vi "FileSaveFile.vi"(0 "VISA IN":refnum<visa-resource-name>, 5 "error in":errorcluster) -> (14 "VISA Out":refnum<visa-resource-name>, 19 "error out":errorcluster)   [LabVIEW 2018, in "PNA-X.lvlib"]
uses:
  PNA-X.lvlib
panel:
  in  "Type":string(combo)
  in  "Port numbers":string
  in  "File":string
  in  "Combo Box":string(combo)="CSA"
  in  "Channel":i32=1
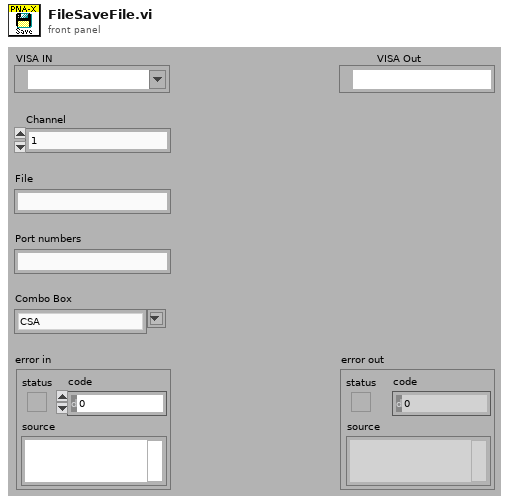
[diagram p1: front panel]
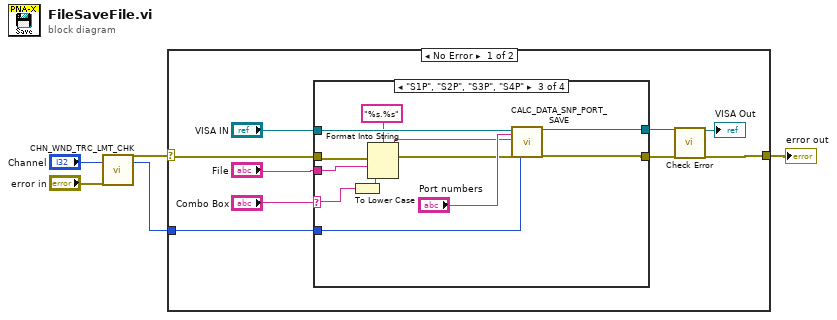
[diagram p0: block diagram]
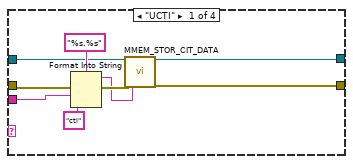
[diagram p2: hidden frame]
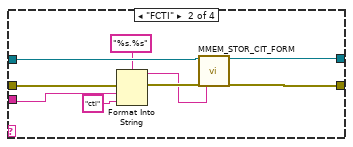
[diagram p3: hidden frame]
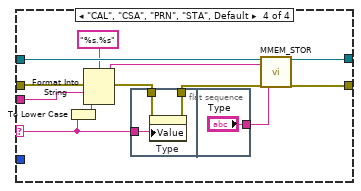
[diagram p4: hidden frame]
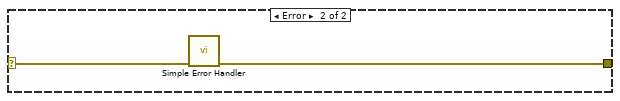
[diagram p5: hidden frame]
diagram:
  n1 = call "CHN_WND_TRC_LMT_CHK.vi"("Channel"="Channel", "error in"="error in") -> ("error out"=w2:errorcluster, "Channel"=w1:i32)  [unwired: 13 in, 3 out]
  n2 = case shown="No Error" w2 {
    selector: w2 -> [w7 w62]
    tunnel: [w14 w61] -> w4
    tunnel: w1 -> [w9 _]
    frame No Error {
      n3 = case shown="\"S1P\", \"S2P\", \"S3P\", \"S4P\"" "Combo Box" {
        selector: "Combo Box" -> [_ _ w33 w47]
        tunnel: w7 -> [w23 w27 w37 w51]
        tunnel: "VISA IN" -> [w17 w31 w43 w55]
        tunnel: [w15 w32 w44 w56] -> w11
        tunnel: [w16 w30 w42 w54] -> w10
        tunnel: w9 -> [_ _ w41 _]
        tunnel: "File" -> [w21 w24 w34 w45]
        frame "UCTI" {
          n4 = Format Into String(format string="%s.%s", error in=w23, w21, "cti" ("input 2")) -> (resulting string=w18:string, error out=w22:errorcluster)  [unwired: 1 in]
          n5 = call "MMEM_STOR_CIT_DATA.vi"("VISA IN"=w17, "error in"=w22, "FileName"=w18) -> ("VISA Out"=w16:refnum<visa-resource-name>, "error out"=w15:errorcluster)  [unwired: 15 in]
        }
        frame "FCTI" {
          n6 = Format Into String(format string="%s.%s", error in=w27, w24, "cti" ("input 2")) -> (resulting string=w25:string, error out=w26:errorcluster)  [unwired: 1 in]
          n7 = call "MMEM_STOR_CIT_FORM.vi"("VISA IN"=w31, "error in"=w26, "FileName"=w25) -> ("VISA Out"=w30:refnum<visa-resource-name>, "error out"=w32:errorcluster)  [unwired: 15 in]
        }
        frame "S1P", "S2P", "S3P", "S4P" {
          n8 = To Lower Case(string=w33) -> (all lower case string=w38:string)
          n9 = Format Into String(format string="%s.%s", error in=w37, w34, w38) -> (resulting string=w35:string, error out=w36:errorcluster)  [unwired: 1 in]
          n10 = call "CALC_DATA_SNP_PORT_SAVE.vi"("VISA IN"=w43, "Port numbers"="Port numbers", "File Path"=w35, "error in"=w36, "Channel"=w41) -> ("VISA Out"=w42:refnum<visa-resource-name>, "error out"=w44:errorcluster)  [unwired: 13 in]
        }
        frame "CAL", "CSA", "PRN", "STA", Default {
          n11 = To Lower Case(string=w47) -> (all lower case string=w46:string)
          n12 = Format Into String(format string="%s.%s", error in=w51, w45, w46) -> (resulting string=w48:string, error out=w50:errorcluster)  [unwired: 1 in]
          n13 = flat-sequence {
            tunnel: w50 -> [w59]
            tunnel: [w58] -> w53
            tunnel: w47 -> [w57]
            tunnel: ["Type"] -> w52
            frame #0 {
              n14 = property on="Type" class="CmbBox"(error in=w59, "Value"=w57) -> (error out=w58:errorcluster)  [unwired: 1 in, 1 out]
            }
            frame #1 {
            }
          }
          n15 = call "MMEM_STOR.vi"("VISA IN"=w55, "File"=w48, "error in"=w53, "Type"=w52) -> ("VISA Out"=w54:refnum<visa-resource-name>, "error out"=w56:errorcluster)  [unwired: 14 in]
        }
      }
      n16 = call "Check Error.vi"("VISA Resource Name"=w10, "error in (no error)"=w11) -> ("dup VISA session"=→"VISA Out":refnum<visa-resource-name>, "error out"=w14:errorcluster)  [unwired: 16 in]
    }
    frame Error {
      n17 = call <vilib>:"Simple Error Handler.vi"("error in (no error)"=w62) -> ("error out"=w61:errorcluster)  [unwired: 4 in, 4 out]
    }
  }
  "error out" <- w4
